vi "emi_Send S&E Error message.vi"(2 "Send(T)":bool=TRUE, 5 "Loop ID in(No Loop)":u16=9999, 9 "error in (no error)":errorcluster, 12 "Var Index":u16, 13 "Elevated priority":bool) -> (6 "Loop ID out":u16, 10 "error out":errorcluster)   [LabVIEW 2011]
doc: "Put error message in the S&E Q. CAn also send if no error, debends exclusively on boolean in."
uses:
  Private/_emi_ S&E Message.ctl
  Private/_emi_ S&E Message type.ctl
  Private/_emi_GFV System ID.vi
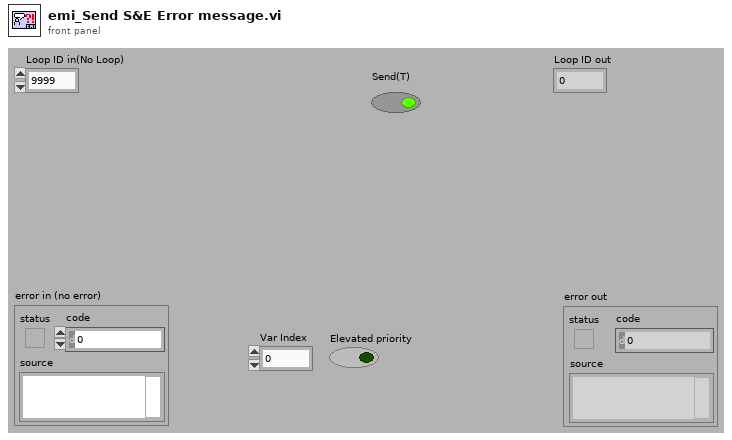
[diagram p1: front panel]
types:
  T1 = typedef "_emi_ S&E Message type.ctl" = enum16{"Error/Warning", "Note", "Debug", "Event", "Alarm Analog", "Alarm Digital", "Annotation"}
  T2 = typedef "_emi_ S&E Message.ctl" = cluster{"Type":T1, "Originate time":dbl, "System":u8, "Loop":u16, "Sub ID":u16, "Elevated priority":bool, "E&S Message content":variant}
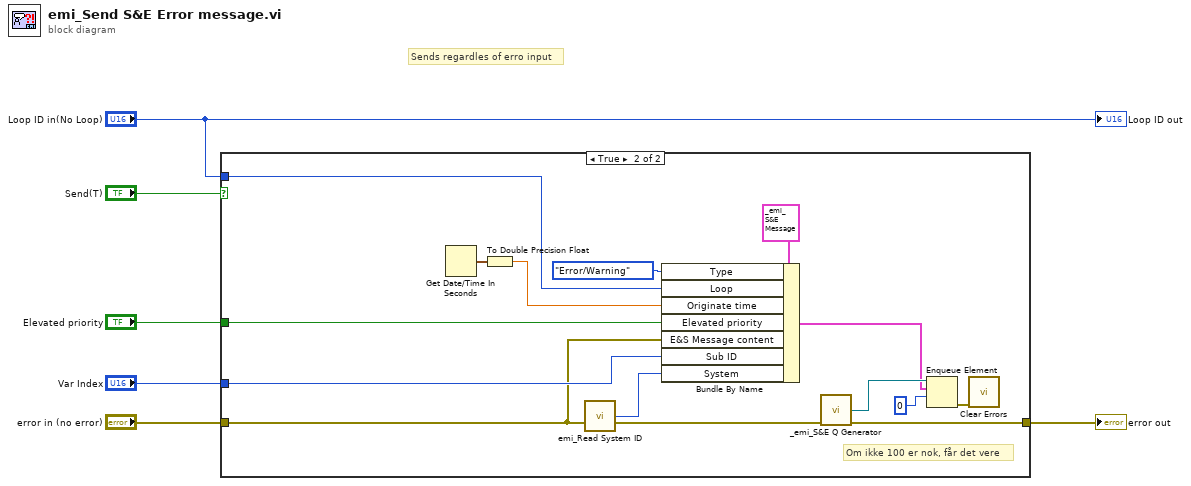
[diagram p0: block diagram]
diagram:
  # "Sends regardles of erro input"
  n1 = case shown="True" "Send(T)" {
    tunnel: "Loop ID in(No Loop)" -> [_ w18]
    tunnel: "Elevated priority" -> [_ w19]
    tunnel: "error in (no error)" -> [w7 w10]
    tunnel: [w7 w16] -> w3
    tunnel: "Var Index" -> [_ w12]
    frame False {
    }
    frame True {
      # "Om ikke 100 er nok, får det vere"
      n2 = Get Date/Time In Seconds() -> (seconds since 1Jan1904=w20:timestamp)
      n3 = To Double Precision Float(number=w20) -> (double precision float=w21:dbl)
      n4 = call "emi_Read System ID.vi"("error in (no error)"=w10) -> ("System ID"=w8:u8, "error out"=w9:errorcluster)  [unwired: 13 in]
      n5 = Bundle By Name(cluster=T2 {"Type"=enum."Error/Warning", "Originate time"=0.0, "System"=0, "Loop"=0, "Sub ID"=0, "Elevated priority"=FALSE, "E&S Message content"=variant} ("E&S Message"), "Type"=_emi__S&E_Message_type."Error/Warning", "Loop"=w18, "Originate time"=w21, "Elevated priority"=w19, "E&S Message content"=w10, "Sub ID"=w12, "System"=w8) -> (w14:T2)
      n6 = call "_emi_S&E Q Generator.vi"("error in (no error)"=w9) -> ("E&S Message Q"=w15:refnum<queue>, "error out"=w16:errorcluster)  [unwired: 13 in]
      n7 = Enqueue Element(queue=w15, element=w14, timeout in ms (-1)=0) -> (error out=w11:errorcluster)  [unwired: 1 in, 2 out]
      n8 = call <vilib>:"Clear Errors.vi"("error in (no error)"=w11) -> ()  [unwired: 6 in, 1 out]
    }
  }
  "error out" <- w3
  "Loop ID out" <- "Loop ID in(No Loop)"
